vi "Receive Device Information.vi"(8 "error in (no error)":errorcluster, 11 "Tovey9150 in":refnum<class "Tovey 9150.lvclass">) -> (0 "error out":errorcluster, 3 "Tovey9150 out":refnum<class "Tovey 9150.lvclass">)   [LabVIEW 2015, in "Tovey 9150.lvclass"]
uses:
  Tovey 9150.lvclass
  Tovey 9150.lvclass/Tovey 9150.ctl
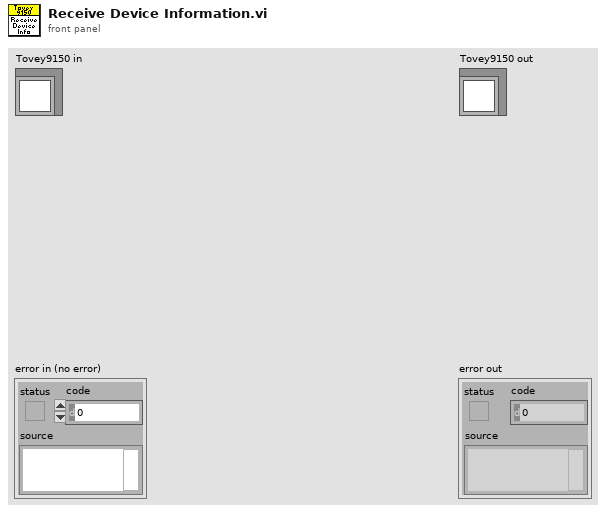
[diagram p1: front panel]
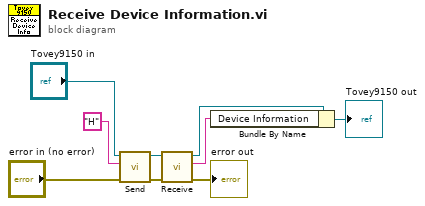
[diagram p0: block diagram]
diagram:
  n1 = call "Send.vi"("error in (no error)"="error in (no error)", "Message"="H", "Tovey9150 in"="Tovey9150 in") -> ("error out"=w4:errorcluster, "Tovey9150 out"=w6:refnum<class "Tovey 9150.lvclass">)  [unwired: 7 in]
  n2 = call "Receive.vi"("error in (no error)"=w4, "Tovey9150 in"=w6) -> ("error out"=→"error out":errorcluster, "Response"=w8:string, "Tovey9150 out"=w5:refnum<class "Tovey 9150.lvclass">)  [unwired: 7 in]
  n3 = Bundle By Name(cluster=w5, "Device Information"=w8) -> (→"Tovey9150 out":refnum<class "Tovey 9150.lvclass">)
